vi "Tuberías.vi"() -> ()   [LabVIEW 2018]
panel:
  out "SD":bool
  out "SC":bool
  out "SB":bool
  out "SA":bool
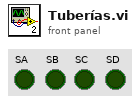
[diagram p1: front panel]
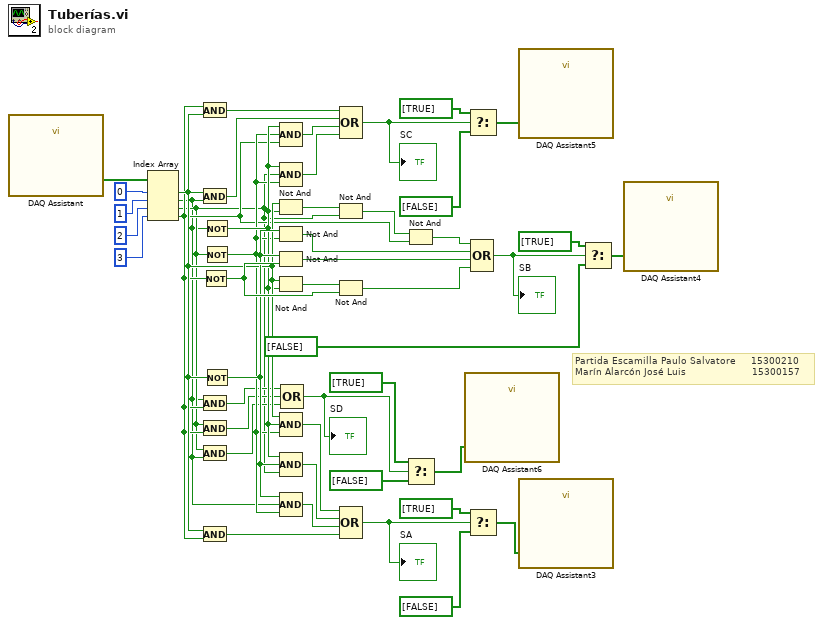
[diagram p0: block diagram]
diagram:
  # "Partida Escamilla Paulo Salvatore     15300210\nMarín Alarcón José Luis                      15300157"
  n1 = call "DAQ Assistant"() -> ("data"=w45:bool[])  [unwired: 17 in, 2 out]
  n2 = Index Array(array=w45, index #1=0 ("index"), index #2=1 ("index"), index #3=2 ("index"), index #4=3 ("index")) -> (element #1=w26:bool, element #2=w16:bool, element #3=w17:bool, element #4=w21:bool)
  n3 = And(x=w21, y=w26) -> (x .and. y?=w27:bool)
  n4 = And(x=w26, y=w16) -> (x .and. y?=w25:bool)
  n5 = And(x=w16, y=w21) -> (x .and. y?=w19:bool)
  n6 = And(x=w17, y=w21) -> (x .and. y?=w20:bool)
  n7 = And(x=w17, y=w16) -> (x .and. y?=w18:bool)
  n8 = And(x=w26, y=w21) -> (x .and. y?=w40:bool)
  n9 = Not(x=w21) -> (.not. x?=w35:bool)
  n10 = Not(x=w16) -> (.not. x?=w23:bool)
  n11 = Not(x=w17) -> (.not. x?=w22:bool)
  n12 = Not(x=w26) -> (.not. x?=w32:bool)
  n13 = Not And(1:w23, 2:w26) -> (0:w30:bool)
  n14 = Not And(1:w22, 2:w32) -> (0:w31:bool)
  n15 = Not And(1:w35, 2:w32) -> (0:w33:bool)
  n16 = Not And(1:w23, 2:w26) -> (0:w36:bool)
  n17 = Compound Arithmetic op=AND(w23, w22, w21) -> (w24:bool)
  n18 = Compound Arithmetic op=AND(w23, w17, w22) -> (w1:bool)
  n19 = Compound Arithmetic op=AND(w26, w23, w22) -> (w37:bool)
  n20 = Compound Arithmetic op=AND(w23, w32, w17) -> (w38:bool)
  n21 = Compound Arithmetic op=AND(w32, w16, w22) -> (w39:bool)
  n22 = Compound Arithmetic op=OR(w19, w20, w18) -> (w3:bool)
  "SD" <- w3
  n23 = Not And(1:w17, 2:w30) -> (0:w29:bool)
  n24 = Not And(1:w35, 2:w36) -> (0:w34:bool)
  n25 = Compound Arithmetic op=OR(w27, w25, w24, w1) -> (w7:bool)
  "SC" <- w7
  n26 = Compound Arithmetic op=OR(w37, w38, w39, w40) -> (w15:bool)
  "SA" <- w15
  n27 = Not And(1:w21, 2:w29) -> (0:w28:bool)
  n28 = Select(t=bool[] [TRUE] ("data"), s=w3, f=bool[] [FALSE] ("data")) -> (s? t:f=w46:bool[])
  n29 = call "DAQ Assistant6"("data"=w46) -> ()  [unwired: 17 in, 2 out]
  n30 = Select(t=bool[] [TRUE] ("data"), s=w7, f=bool[] [FALSE] ("data")) -> (s? t:f=w4:bool[])
  n31 = Select(t=bool[] [TRUE] ("data"), s=w15, f=bool[] [FALSE] ("data")) -> (s? t:f=w12:bool[])
  n32 = Compound Arithmetic op=OR(w28, w31, w33, w34) -> (w11:bool)
  "SB" <- w11
  n33 = call "DAQ Assistant5"("data"=w4) -> ()  [unwired: 17 in, 2 out]
  n34 = call "DAQ Assistant3"("data"=w12) -> ()  [unwired: 17 in, 2 out]
  n35 = Select(t=bool[] [TRUE] ("data"), s=w11, f=bool[] [FALSE] ("data")) -> (s? t:f=w8:bool[])
  n36 = call "DAQ Assistant4"("data"=w8) -> ()  [unwired: 17 in, 2 out]
